vi "Configure.vi"(8 "error in (no error)":errorcluster, 10 "Msg in":T1, 11 "FakePressureController in":refnum<class "MagAnalysis_Online.lvclass">) -> (0 "error out":errorcluster, 1 "new command":string, 2 "Msg out":T1, 3 "FakePressureController out":refnum<class "MagAnalysis_Online.lvclass">)   [LabVIEW 2011, in "MagAnalysis_Online.lvclass"]
uses:
  MagAnalysis_Online.lvclass
  DriverMsg.ctl
  MagAnalysis_Online.lvclass/MagAnalysis_Online.ctl
  OnOffTypeDef.ctl
  BaseDriver/BaseDriver.lvclass
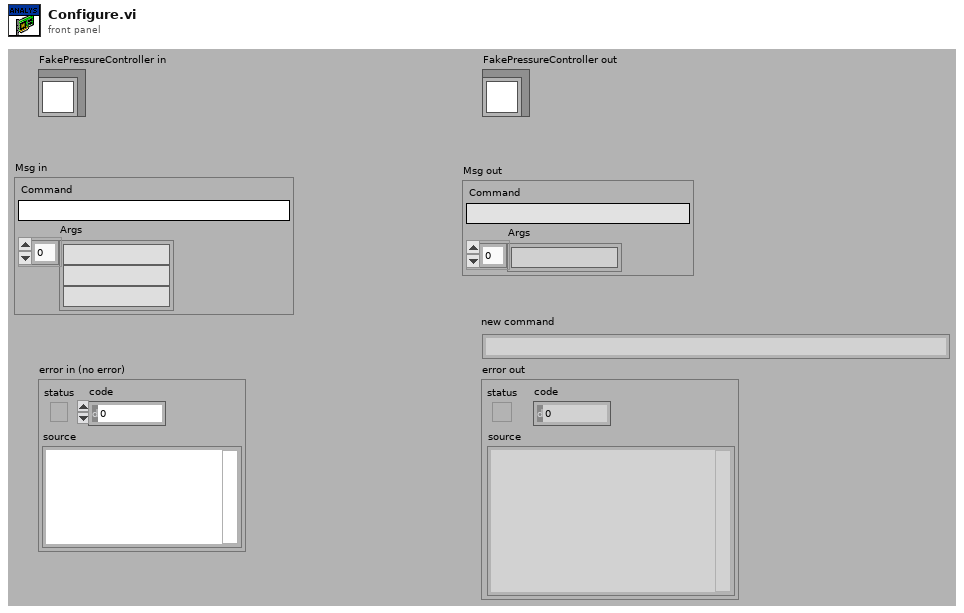
[diagram p1: front panel]
types:
  T1 = typedef "DriverMsg.ctl" = cluster{"Command":string, "Args":string[]}
  T2 = typedef "OnOffTypeDef.ctl" = enum16{"off", "on"}
  T3 = typedef "MagAnalysis_Online.lvclass/settings_TypDef.ctl" = cluster{"CamSettings":T4, "timeout":T7, "Screws":T8, "number of cam":dbl, "X size":dbl, "srewstart":T11, "Save":T2, "offset":dbl, "localsavingpath":path}
  T4 = typedef "CamSettings_Typdef.ctl" = cluster{"Cam 0":T5, "Cam 1":T5, "Cam 2":T5, "Cam 3":T5}
  T5 = typedef "CamSettingSUB_TypDEf.ctl" = cluster{"position":dbl, "Field of view":dbl, "start":dbl, "end":dbl, "center":dbl, "Lens":T6, "Forward":T2, "Spec_Calib_file 2":path, "map":path, "y size":i32}
  T6 = typedef "CamAndObj_TypDEf.ctl" = enum16{"FL1-f8x08", "FL1-f8x06", "FL1-f8", "ch300-f50", "FL2G-f8", "FL3M14-f8", "FL3M14-f8x08", "FL3M14-f8x08(2x2)"}
  T7 = typedef "numericVariable_TypeDef.ctl" = cluster{"Value":dbl, "Min":dbl, "Max":dbl, "StepSize":dbl, "Tolerance":dbl, "valueactual":dbl}
  T8 = typedef "SrewMaster_TYpDef.ctl" = cluster{"Cam 0":T9, "Cam 1":T9, "Cam 2":T9, "Cam 3":T9}
  T9 = typedef "srew_TypDEf.ctl" = cluster{"S 0":T10, "S 1":T10, "S 2":T10, "S 3":T10, "S 4":T10, "S 5":T10}
  T10 = typedef "ScrewSub_Typdef.ctl" = cluster{"0":i32, "1":i32, "2":i32, "3":i32}
  T11 = typedef "screwstart.ctl" = cluster{"Cam 0":dbl, "Cam 1":dbl, "Cam 2":dbl, "Cam 3":dbl}
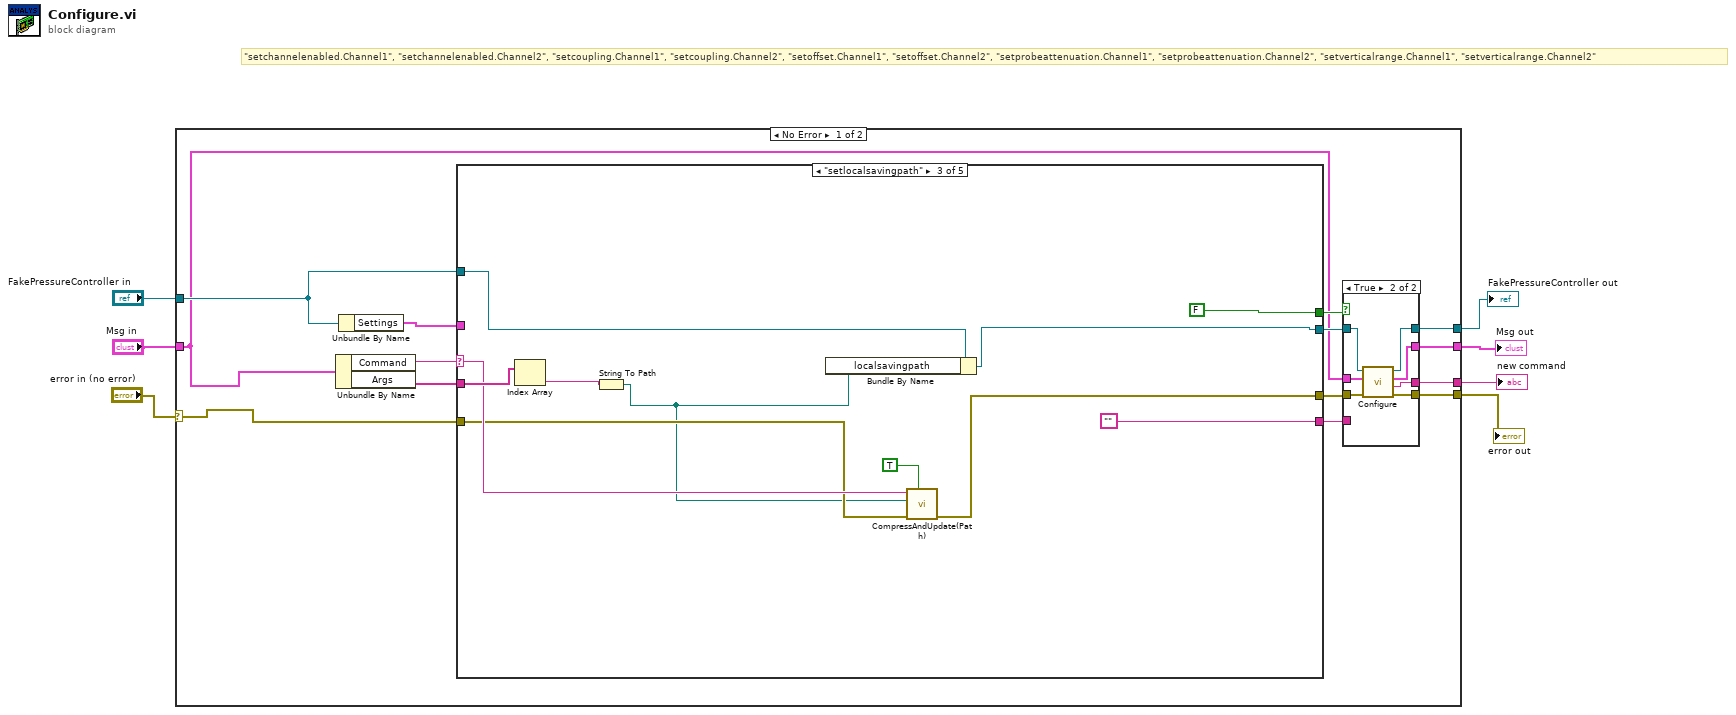
[diagram p0: block diagram]
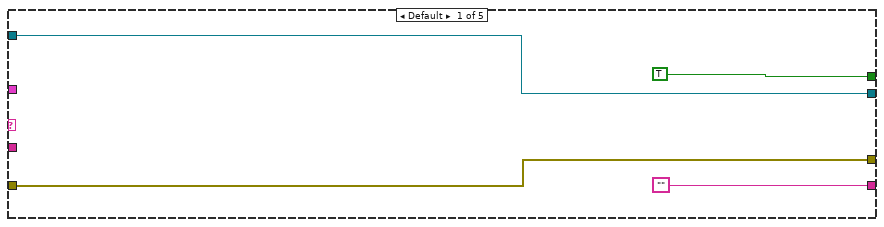
[diagram p3: hidden frame]
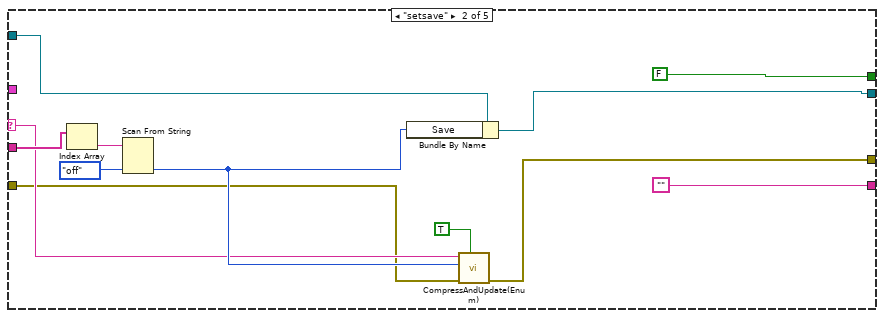
[diagram p4: hidden frame]
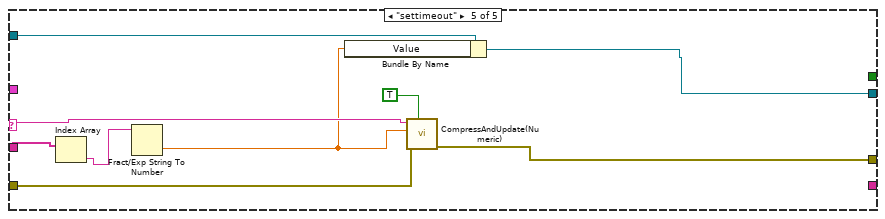
[diagram p6: hidden frame]
diagram:
  # "\"setchannelenabled.Channel1\", \"setchannelenabled.Channel2\", \"setcoupling.Channel1\", \"setcoupling.Channel2\", \"setoffset.Channel1\", \"setoffset.Channel2\", \"setprobeattenuation.Channel1\", \"setprobeattenuation.Channel2\", \"setverticalrange.Channel1\", \"setverticalrange.Channel2\""
  n1 = case shown="No Error" "error in (no error)" {
    selector: "error in (no error)" -> [w8 w73]
    tunnel: "FakePressureController in" -> [w12 w71]
    tunnel: [w20 w71] -> w4
    tunnel: [w18 w73] -> w1
    tunnel: "Msg in" -> [w9 w72]
    tunnel: [w16 w72] -> w3
    tunnel: [w14 _] -> w2
    frame No Error {
      n2 = Unbundle By Name(w9) -> ("Command"=w13:string, "Args"=w10:string[])
      n3 = Unbundle By Name(w12) -> ("Settings"=w11:T3)
      n4 = case shown="\"setlocalsavingpath\"" w13 {
        selector: w13 -> [_ w39 w54 _ w65]
        tunnel: w8 -> [w35 w38 w53 w60 w63]
        tunnel: w10 -> [_ w46 w58 _ w70]
        tunnel: w12 -> [w36 w43 w57 w61 w68]
        tunnel: [w36 w42 w56 w61 w67] -> w21
        tunnel: ["" ("Complete") "" ("Complete") "" ("Complete") _ _] -> w15
        tunnel: [w35 w37 w52 w60 w62] -> w19
        tunnel: [TRUE FALSE FALSE _ _] -> w17
        tunnel: w11 -> [_ _ _ _ _]
        frame Default {
        }
        frame "setsave" {
          n5 = Index Array(array=w46) -> (element=w45:string)  [unwired: 1 in]
          n6 = Scan From String(input string=w45, default 1=OnOffTypeDef."off" ("Save")) -> (output 1=w40:T2)  [unwired: 3 in, 3 out]
          n7 = Bundle By Name(cluster=w43, "Save"=w40) -> (w42:refnum<class "MagAnalysis_Online.lvclass">)
          n8 = call "CompressAndUpdate(Enum).vi"("force CVT update (false)"=TRUE, "error in"=w38, "enum variant"=w40, "command or variable name"=w39) -> ("error out"=w37:errorcluster)  [unwired: 7 in]
        }
        frame "setlocalsavingpath" {
          n9 = Index Array(array=w58) -> (element=w51:string)  [unwired: 1 in]
          n10 = String To Path(string=w51) -> (path=w50:path)
          n11 = Bundle By Name(cluster=w57, "localsavingpath"=w50) -> (w56:refnum<class "MagAnalysis_Online.lvclass">)
          n12 = call "CompressAndUpdate(Path).vi"("force CVT update (false)"=TRUE, "error in"=w53, "Path"=w50, "command or variable name"=w54) -> ("error out"=w52:errorcluster)  [unwired: 7 in]
        }
        frame "Abort" {
        }
        frame "settimeout" {
          n13 = Index Array(array=w70) -> (element=w69:string)  [unwired: 1 in]
          n14 = Fract/Exp String To Number(string=w69) -> (number=w64:dbl)  [unwired: 3 in, 1 out]
          n15 = Bundle By Name(cluster=w68, "Value"=w64) -> (w67:refnum<class "MagAnalysis_Online.lvclass">)
          n16 = call "CompressAndUpdate(Numeric).vi"("force CVT update (false)"=TRUE, "error in"=w63, "Numeric"=w64, "command or variable name"=w65) -> ("error out"=w62:errorcluster)  [unwired: 7 in]
        }
      }
      n17 = case shown="True" w17 {
        tunnel: w21 -> [w23 w32]
        tunnel: [w23 w31] -> w20
        tunnel: [w24 w30] -> w14
        tunnel: w19 -> [w22 w29]
        tunnel: [w22 w28] -> w18
        tunnel: w9 -> [w25 w27]
        tunnel: [w25 w26] -> w16
        tunnel: w15 -> [w24 _]
        frame False {
        }
        frame True {
          n18 = call-parent "Configure.vi"("error in (no error)"=w29, "Msg in"=w27, "BaseDriver in"=w32) -> ("error out"=w28:errorcluster, "new command"=w30:string, "Msg out"=w26:T1, "BaseDriver out"=w31:refnum<class "MagAnalysis_Online.lvclass">)  [unwired: 5 in]
        }
      }
    }
    frame Error {
    }
  }
  "error out" <- w1
  "FakePressureController out" <- w4
  "new command" <- w2
  "Msg out" <- w3
